vi "shooter control.vi"(0 "Back Shooter DevRef In":T1={"DeviceStatus"={"status"=FALSE, "code"=0, "source"=""}, "Type"=enum."PWM", "PWM"={"Digital Module"=enum."Digital Module 2", "PWM Channel"=enum."PWM 1", "DeadBand"={"Name"="", "maxPositivePwm"=0, "minPositivePwm"=0, "centerPwm"=0, "maxNegativePwm"=0, "minNegativePwm"=0, "angularRange"=0}}, "CAN"={"Device Number"=0, "Control Mode"=enum."Percent VBus", "Semaphore"=refnum, "Max Vout"=12.0}, "Invert"=FALSE, "TransformRef"=refnum, "InvTransformRef"=refnum}, 1 "Front Shooter DevRef In":T1={"DeviceStatus"={"status"=FALSE, "code"=0, "source"=""}, "Type"=enum."PWM", "PWM"={"Digital Module"=enum."Digital Module 2", "PWM Channel"=enum."PWM 1", "DeadBand"={"Name"="", "maxPositivePwm"=0, "minPositivePwm"=0, "centerPwm"=0, "maxNegativePwm"=0, "minNegativePwm"=0, "angularRange"=0}}, "CAN"={"Device Number"=0, "Control Mode"=enum."Percent VBus", "Semaphore"=refnum, "Max Vout"=12.0}, "Invert"=FALSE, "TransformRef"=refnum, "InvTransformRef"=refnum}, 5 "Closed Loop On/Off":bool, 7 "Power On/Off":bool, 9 "Joystick Throttle":dbl, 11 "Manual Control":bool, 12 "Distance":dbl) -> (3 "Front Shooter DevRef Out":T1={"DeviceStatus"={"status"=FALSE, "code"=0, "source"=""}, "Type"=enum."PWM", "PWM"={"Digital Module"=enum."Digital Module 2", "PWM Channel"=enum."PWM 1", "DeadBand"={"Name"="", "maxPositivePwm"=0, "minPositivePwm"=0, "centerPwm"=0, "maxNegativePwm"=0, "minNegativePwm"=0, "angularRange"=0}}, "CAN"={"Device Number"=0, "Control Mode"=enum."Percent VBus", "Semaphore"=refnum, "Max Vout"=12.0}, "Invert"=FALSE, "TransformRef"=refnum, "InvTransformRef"=refnum}, 4 "Back Shooter DevRef Out":T1={"DeviceStatus"={"status"=FALSE, "code"=0, "source"=""}, "Type"=enum."PWM", "PWM"={"Digital Module"=enum."Digital Module 2", "PWM Channel"=enum."PWM 1", "DeadBand"={"Name"="", "maxPositivePwm"=0, "minPositivePwm"=0, "centerPwm"=0, "maxNegativePwm"=0, "minNegativePwm"=0, "angularRange"=0}}, "CAN"={"Device Number"=0, "Control Mode"=enum."Percent VBus", "Semaphore"=refnum, "Max Vout"=12.0}, "Invert"=FALSE, "TransformRef"=refnum, "InvTransformRef"=refnum}, 6 "FrontShooterOut":dbl, 8 "BackShooterOut":dbl)   [LabVIEW 2012]
uses:
  <vilib>/Rock Robotics/WPI/MotorControl/WPI_MotorControlDeviceRef.ctl
  <vilib>/Rock Robotics/SystemInterfaces/Typedef/FPGA_TypedefDigitalModule.ctl
  <vilib>/Rock Robotics/SystemInterfaces/DIO/FPGA_DIOPWMChannel.ctl
  <vilib>/Rock Robotics/WPI/PWM/WPI_PWMDeadband.ctl
  <vilib>/Rock Robotics/WPI/CAN/Jaguar/SubVIs/WPI_CANJaguar_ControlMode.ctl
  <vilib>/Rock Robotics/WPI/PWM/WPI_PWMTransform_ConPane.ctl
  <vilib>/Rock Robotics/WPI/CAN/Jaguar/SubVIs/WPI_CANJaguar_SpeedReference.ctl
  Robot Global Data.vi
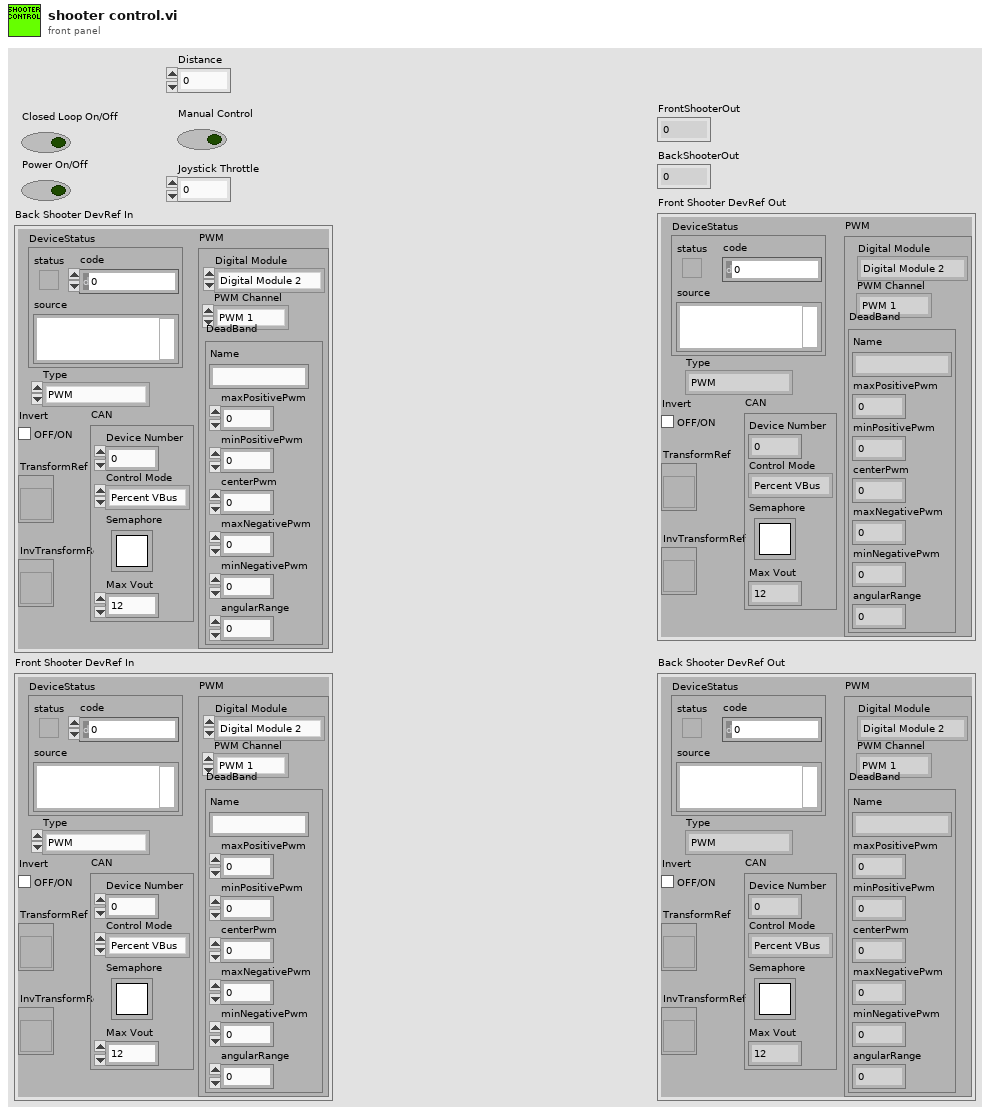
[diagram p1: front panel]
types:
  T1 = typedef "WPI_MotorControlDeviceRef.ctl" = cluster{"DeviceStatus":errorcluster, "Type":enum16{"PWM", "CAN"}, "PWM":cluster{"Digital Module":T2, "PWM Channel":T3, "DeadBand":T4}, "CAN":cluster{"Device Number":u8, "Control Mode":T5, "Semaphore":T6, "Max Vout":dbl}, "Invert":bool, "TransformRef":T7, "InvTransformRef":T7}
  T2 = typedef "FPGA_TypedefDigitalModule.ctl" = enum16{"Digital Module 1", "Digital Module 2"}
  T3 = typedef "FPGA_DIOPWMChannel.ctl" = enum8{"PWM 1", "PWM 2", "PWM 3", "PWM 4", "PWM 5", "PWM 6", "PWM 7", "PWM 8", "PWM 9", "PWM 10", "Invalid"}
  T4 = typedef "WPI_PWMDeadband.ctl" = cluster{"Name":string, "maxPositivePwm":i32, "minPositivePwm":i32, "centerPwm":i32, "maxNegativePwm":i32, "minNegativePwm":i32, "angularRange":u16}
  T5 = typedef "WPI_CANJaguar_ControlMode.ctl" = enum8{"Percent VBus", "Current", "Speed", "Position", "Voltage"}
  T6 = typedef "Semaphore RefNum" = refnum<k1>
  T7 = typedef "WPI_PWMTransform_ConPane.ctl" = refnum<vi>
  T8 = typedef "WPI_CANJaguar_SpeedReference.ctl" = u8
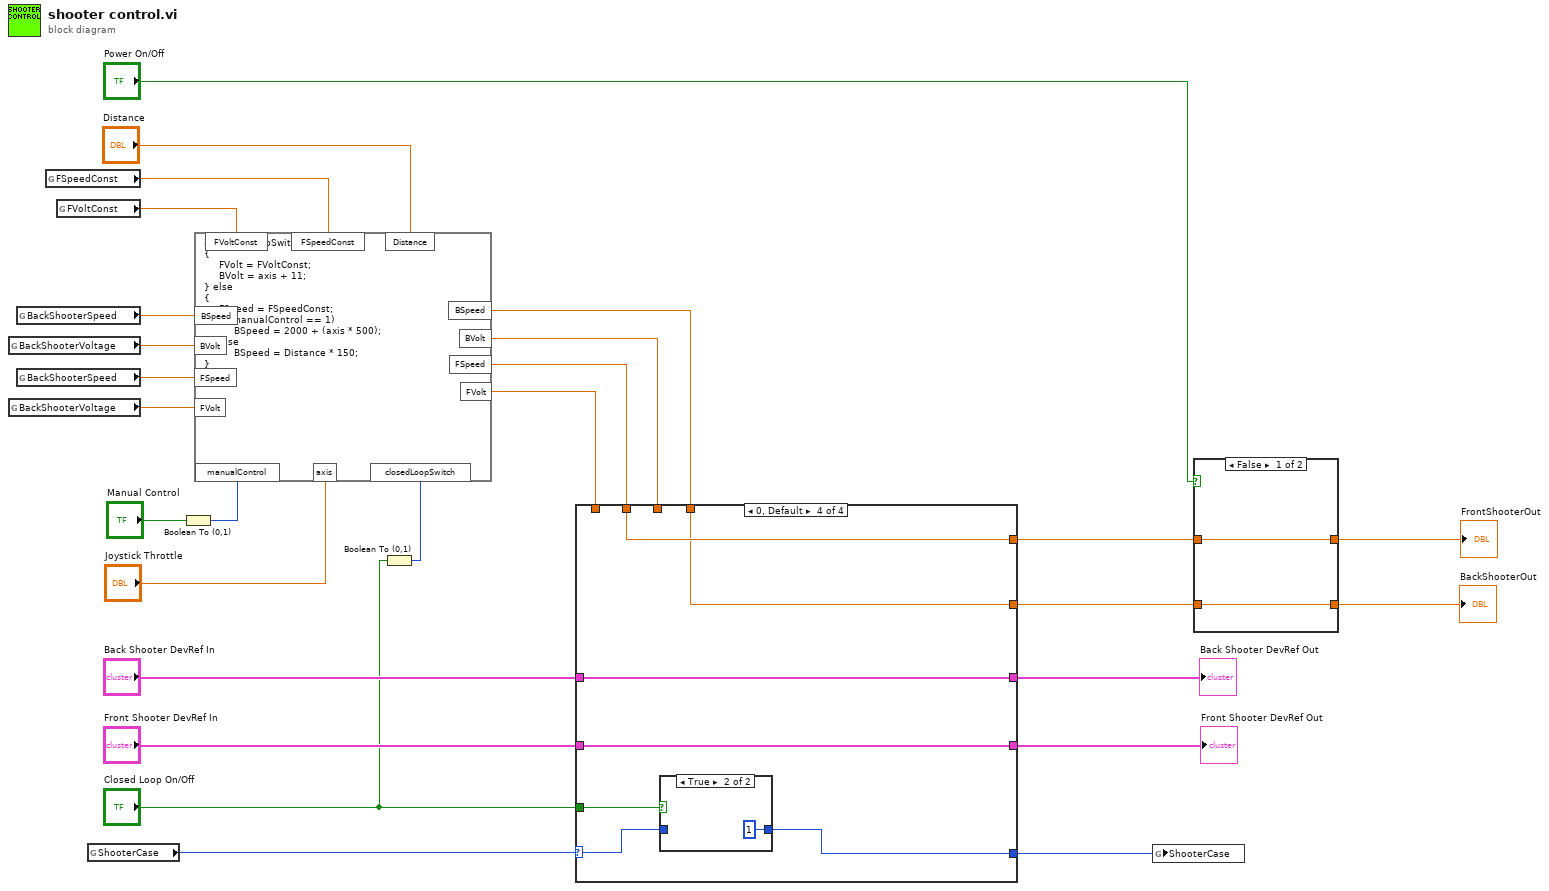
[diagram p0: block diagram]
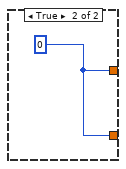
[diagram p2: hidden frame]
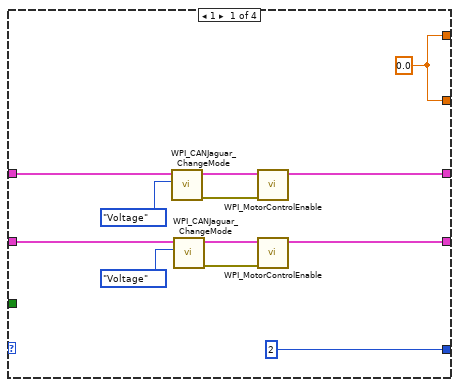
[diagram p3: hidden frame]
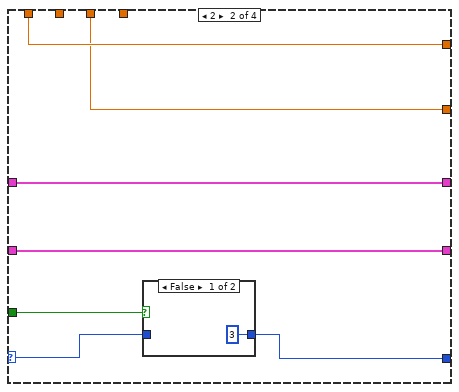
[diagram p4: hidden frame]
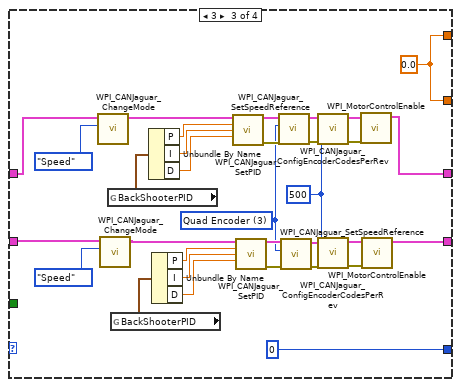
[diagram p6: hidden frame]
diagram:
  n1 = global read "Robot Global Data.vi" "BackShooterVoltage"() -> (w20:dbl)
  n2 = global read "Robot Global Data.vi" "BackShooterVoltage"() -> (w18:dbl)
  n3 = global read "Robot Global Data.vi" "BackShooterSpeed"() -> (w21:dbl)
  n4 = global read "Robot Global Data.vi" "BackShooterSpeed"() -> (w19:dbl)
  n5 = global read "Robot Global Data.vi" "FSpeedConst"() -> (w6:dbl)
  n6 = global read "Robot Global Data.vi" "FVoltConst"() -> (w5:dbl)
  n7 = global read "Robot Global Data.vi" "ShooterCase"() -> (w23:i8)
  n8 = Boolean To (0,1)(Boolean="Manual Control") -> (0, 1=w2:i16)
  n9 = Boolean To (0,1)(Boolean="Closed Loop On/Off") -> (0, 1=w3:i16)
  n10 = formula code="if (closedLoopSwitch == 1)\n{\n     FVolt = FVoltConst;\n     BVolt = axis + 11;\n} else\n{\n     FSpeed = FSpeedConst;\n     if (manualControl == 1)\n          BSpeed = 2000 + (axis * 500);\n     else\n          BSpeed = Distance * 150;\n}"("BSpeed"=w21, "BVolt"=w20, "FSpeed"=w19, "FVolt"=w18, "closedLoopSwitch"=w3, "axis"="Joystick Throttle", "FVoltConst"=w5, "FSpeedConst"=w6, "manualControl"=w2, "Distance"="Distance") -> ("BSpeed"=w9:dbl, "BVolt"=w10:dbl, "FSpeed"=w11:dbl, "FVolt"=w12:dbl)
  n11 = case shown="0, Default" w23 {
    selector: w23 -> [_ w43 _ w83]
    tunnel: [i8 2 ("ShooterCase") w42 i8 0 ("ShooterCase") w84] -> w22
    tunnel: "Back Shooter DevRef In" -> [w38 w46 w78 w87]
    tunnel: "Front Shooter DevRef In" -> [w37 w45 w77 w86]
    tunnel: [w30 w46 w50 w87] -> w25
    tunnel: [w29 w45 w51 w86] -> w24
    tunnel: "Closed Loop On/Off" -> [_ w44 _ w85]
    tunnel: w12 -> [_ w41 _ _]
    tunnel: w11 -> [_ _ _ w82]
    tunnel: w10 -> [_ w40 _ _]
    tunnel: w9 -> [_ _ _ w81]
    tunnel: [w28 w41 w49 w82] -> w8
    tunnel: [w28 w40 w49 w81] -> w7
    frame 1 {
      w28 = 0.0 ("FSpeed")
      n12 = call <vilib>:"WPI_CANJaguar_ChangeMode.vi"("Control Mode"=WPI_CANJaguar_ControlMode."Voltage", "CAN Jaguar Ref"=w38) -> ("error out"=w31:errorcluster, "CAN Jaguar Ref Out"=w32:T1)  [unwired: 8 in]
      n13 = call <vilib>:"WPI_CANJaguar_ChangeMode.vi"("Control Mode"=WPI_CANJaguar_ControlMode."Voltage", "CAN Jaguar Ref"=w37) -> ("error out"=w33:errorcluster, "CAN Jaguar Ref Out"=w34:T1)  [unwired: 8 in]
      n14 = call <vilib>:"WPI_MotorControlEnable.vi"("error in (no error)"=w31, "CAN Jaguar Ref"=w32) -> ("CAN Jaguar Ref Out"=w30:T1)  [unwired: 8 in, 1 out]
      n15 = call <vilib>:"WPI_MotorControlEnable.vi"("error in (no error)"=w33, "CAN Jaguar Ref"=w34) -> ("CAN Jaguar Ref Out"=w29:T1)  [unwired: 8 in, 1 out]
    }
    frame 2 {
      n16 = case shown="False" w44 {
        tunnel: [i8 3 ("ShooterCase") w48] -> w42
        tunnel: w43 -> [_ w48]
        frame False {
        }
        frame True {
        }
      }
    }
    frame 3 {
      w49 = 0.0 ("FSpeed")
      w56 = u16 500 ("Encoder Codes Per Rev")
      w61 = T8 3 items=["Encoder"=0, "Inv Encoder"=2, "Quad Encoder"=3, "None"=255] ("Speed Reference")
      n17 = call <vilib>:"WPI_CANJaguar_ChangeMode.vi"("Control Mode"=WPI_CANJaguar_ControlMode."Speed", "CAN Jaguar Ref"=w78) -> ("CAN Jaguar Ref Out"=w76:T1)  [unwired: 8 in, 1 out]
      n18 = call <vilib>:"WPI_CANJaguar_ChangeMode.vi"("Control Mode"=WPI_CANJaguar_ControlMode."Speed", "CAN Jaguar Ref"=w77) -> ("CAN Jaguar Ref Out"=w67:T1)  [unwired: 8 in, 1 out]
      n19 = global read "Robot Global Data.vi" "BackShooterPID"() -> (w75:cluster{"P":dbl, "I":dbl, "D":dbl})
      n20 = global read "Robot Global Data.vi" "BackShooterPID"() -> (w71:cluster{"P":dbl, "I":dbl, "D":dbl})
      n21 = Unbundle By Name(w75) -> ("P"=w74:dbl, "I"=w73:dbl, "D"=w72:dbl)
      n22 = Unbundle By Name(w71) -> ("P"=w70:dbl, "I"=w69:dbl, "D"=w68:dbl)
      n23 = call <vilib>:"WPI_CANJaguar_SetPID.vi"("CAN Jaguar Ref"=w76, "P"=w74, "I"=w73, "D"=w72) -> ("CAN Jaguar Ref Out"=w64:T1, "error out"=w65:errorcluster)  [unwired: 10 in]
      n24 = call <vilib>:"WPI_CANJaguar_SetPID.vi"("CAN Jaguar Ref"=w67, "P"=w70, "I"=w69, "D"=w68) -> ("CAN Jaguar Ref Out"=w63:T1, "error out"=w62:errorcluster)  [unwired: 10 in]
      n25 = call <vilib>:"WPI_CANJaguar_SetSpeedReference.vi"("error in (no error)"=w65, "Speed Reference"=w61, "CAN Jaguar Ref"=w64) -> ("error out"=w60:errorcluster, "CAN Jaguar Ref Out"=w59:T1)  [unwired: 7 in]
      n26 = call <vilib>:"WPI_CANJaguar_SetSpeedReference.vi"("error in (no error)"=w62, "Speed Reference"=w61, "CAN Jaguar Ref"=w63) -> ("error out"=w57:errorcluster, "CAN Jaguar Ref Out"=w58:T1)  [unwired: 7 in]
      n27 = call <vilib>:"WPI_CANJaguar_ConfigEncoderCodesPerRev.vi"("error in (no error)"=w60, "Encoder Codes Per Rev"=w56, "CAN Jaguar Ref"=w59) -> ("error out"=w55:errorcluster, "CAN Jaguar Ref Out"=w54:T1)  [unwired: 7 in]
      n28 = call <vilib>:"WPI_CANJaguar_ConfigEncoderCodesPerRev.vi"("error in (no error)"=w57, "Encoder Codes Per Rev"=w56, "CAN Jaguar Ref"=w58) -> ("error out"=w53:errorcluster, "CAN Jaguar Ref Out"=w52:T1)  [unwired: 7 in]
      n29 = call <vilib>:"WPI_MotorControlEnable.vi"("error in (no error)"=w55, "CAN Jaguar Ref"=w54) -> ("CAN Jaguar Ref Out"=w50:T1)  [unwired: 8 in, 1 out]
      n30 = call <vilib>:"WPI_MotorControlEnable.vi"("error in (no error)"=w53, "CAN Jaguar Ref"=w52) -> ("CAN Jaguar Ref Out"=w51:T1)  [unwired: 8 in, 1 out]
    }
    frame 0, Default {
      n31 = case shown="True" w85 {
        tunnel: [w88 i8 1 ("ShooterCase")] -> w84
        tunnel: w83 -> [w88 _]
        frame False {
        }
        frame True {
        }
      }
    }
  }
  "Front Shooter DevRef Out" <- w24
  "Back Shooter DevRef Out" <- w25
  n32 = global write "Robot Global Data.vi" "ShooterCase"(w22) -> ()
  n33 = case shown="False" "Power On/Off" {
    tunnel: [w91 w92] -> w16
    tunnel: [w90 w92] -> w15
    tunnel: w8 -> [w91 _]
    tunnel: w7 -> [w90 _]
    frame False {
    }
    frame True {
      w92 = 0
    }
  }
  "FrontShooterOut" <- w16
  "BackShooterOut" <- w15
